vi "副屏设置.vi"() -> ()   [LabVIEW 2016, in "副屏.lvlib"]
uses:
  <vilib>/Utility/config.llb/NI_LVConfig.lvlib
panel:
  in  "屏幕类型":enum16{"HDMI屏", "串口屏"}(ring)
  in  "氟化物":bool caption="氨氮禁用"
  in  "ORP":bool caption="氨氮禁用"
  in  "启用副屏":bool=TRUE caption="氨氮禁用"
  in  "关闭":bool
  in  "底部状态栏显示信息":string="一体化微型水质监测系统"
  in  "流速":bool caption="氨氮禁用"
  in  "瞬时流量":bool caption="氨氮禁用"
  in  "湿度":bool=TRUE caption="氨氮禁用"
  in  "水位":bool caption="氨氮禁用"
  in  "室温":bool=TRUE caption="氨氮禁用"
  in  "CODCr":bool caption="氨氮禁用"
  in  "CODMn":bool caption="氨氮禁用"
  in  "总氮":bool caption="氨氮禁用"
  in  "总磷":bool caption="氨氮禁用"
  in  "氨氮":bool caption="氨氮禁用"
  in  "Turb":bool caption="氨氮禁用"
  in  "Cond":bool caption="氨氮禁用"
  in  "DO":bool caption="氨氮禁用"
  in  "pH":bool caption="氨氮禁用"
  in  "水温":bool caption="氨氮禁用"
  # "副屏显示信息设置"
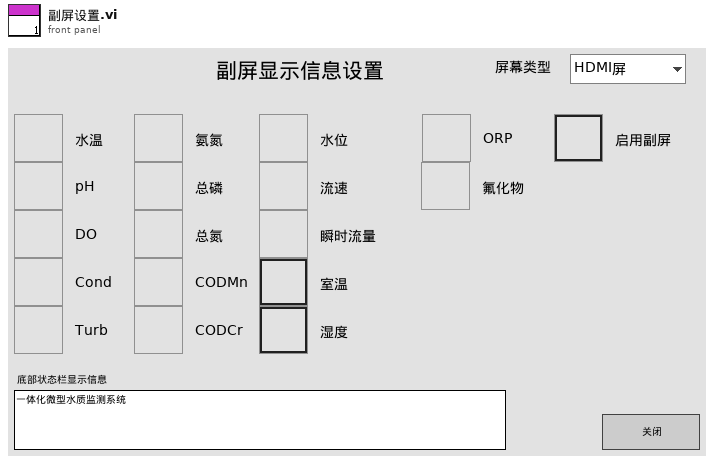
[diagram p1: front panel]
types:
  T1 = typedef "NI_LVConfig.lvlib/Config Data RefNum.ctl" = refnum<k1>
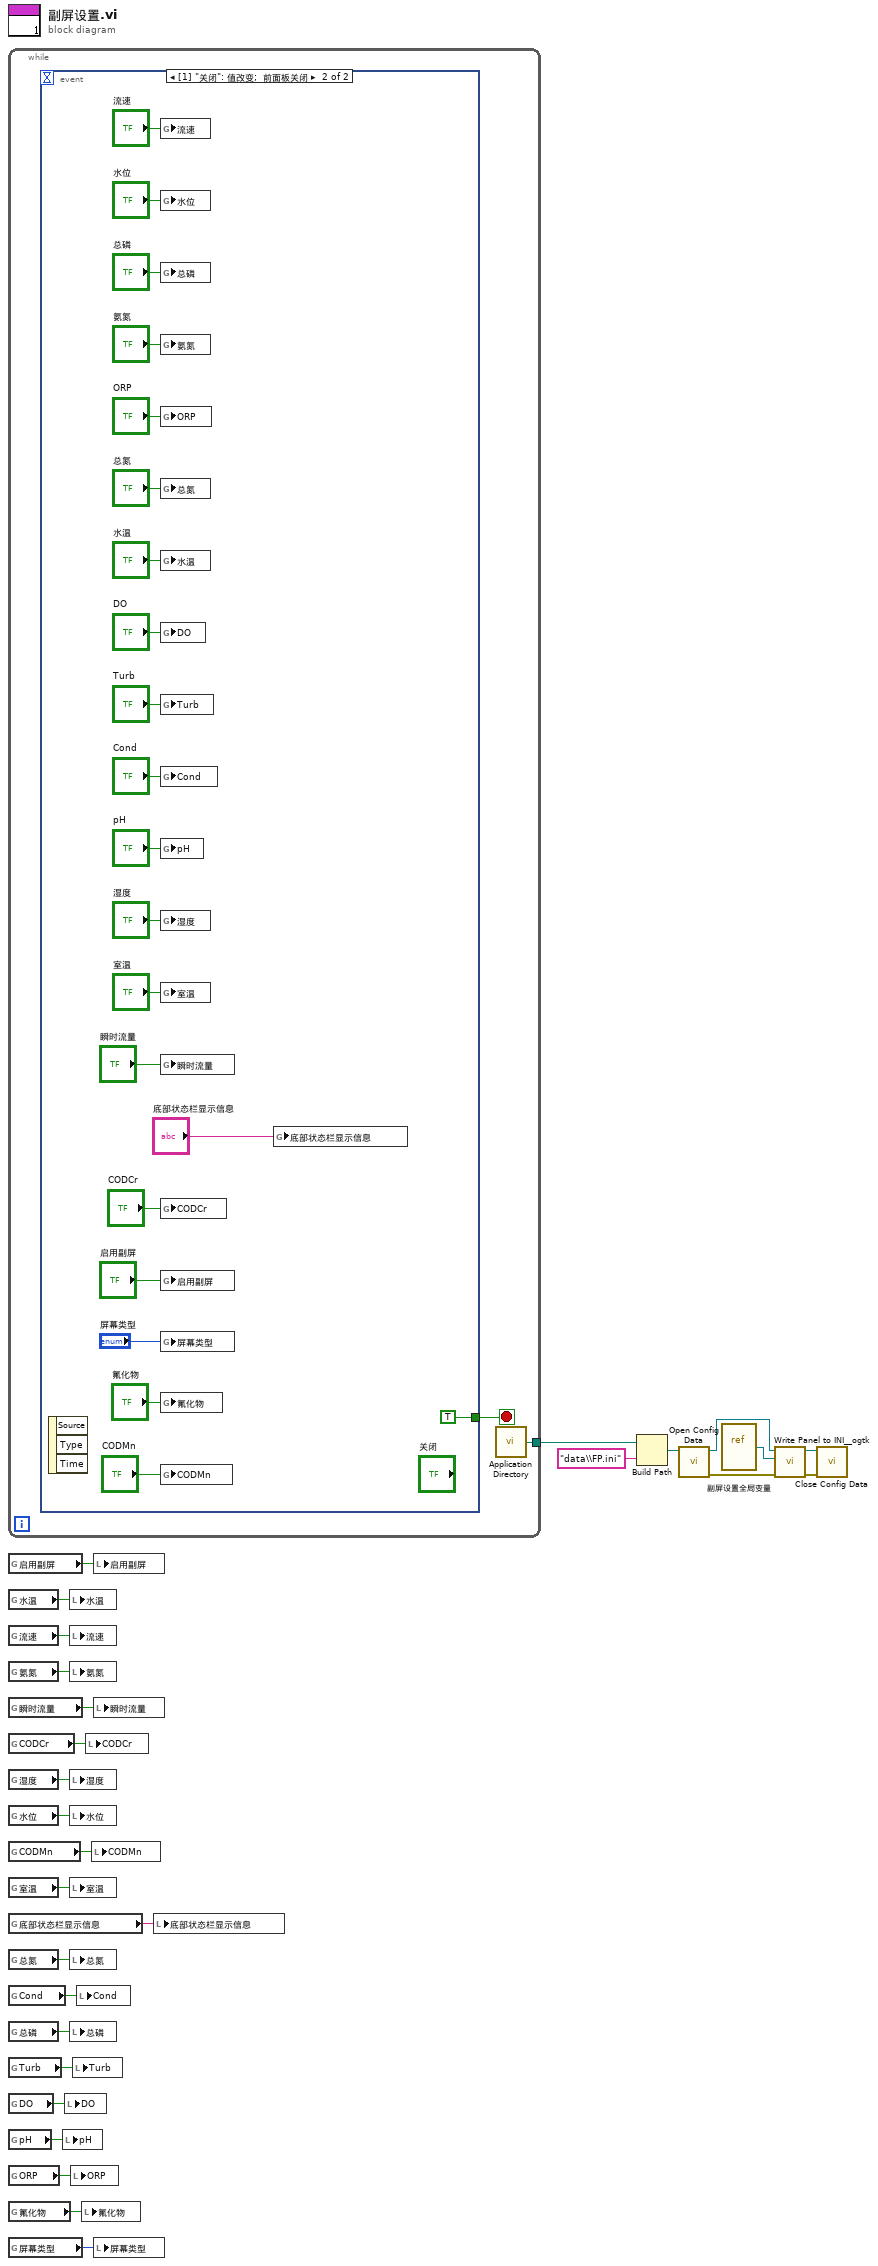
[diagram p0: block diagram]
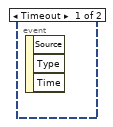
[diagram p2: hidden frame]
diagram:
  n1 = while {
    tunnel: [w29] -> w5
    stop <- w30 stop-if-true
    n2 = event shown="[1] \"关闭\": 值改变;  前面板关闭" {
      selector: _ -> [_ _]
      dyn-events: _ -> [_ _]
      timeout: _ -> [_ _]
      tunnel: [_ TRUE] -> w30
      event Timeout {
        n3 = event-data() -> ()  [unwired: 1 in, 3 out]
      }
      event "关闭": Value Change; Panel Close {
        n4 = event-data() -> ()  [unwired: 1 in, 3 out]
        n5 = global write "副屏设置全局变量.vi" "流速"("流速") -> ()
        n6 = global write "副屏设置全局变量.vi" "水位"("水位") -> ()
        n7 = global write "副屏设置全局变量.vi" "总磷"("总磷") -> ()
        n8 = global write "副屏设置全局变量.vi" "氨氮"("氨氮") -> ()
        n9 = global write "副屏设置全局变量.vi" "ORP"("ORP") -> ()
        n10 = global write "副屏设置全局变量.vi" "总氮"("总氮") -> ()
        n11 = global write "副屏设置全局变量.vi" "水温"("水温") -> ()
        n12 = global write "副屏设置全局变量.vi" "DO"("DO") -> ()
        n13 = global write "副屏设置全局变量.vi" "Turb"("Turb") -> ()
        n14 = global write "副屏设置全局变量.vi" "Cond"("Cond") -> ()
        n15 = global write "副屏设置全局变量.vi" "pH"("pH") -> ()
        n16 = global write "副屏设置全局变量.vi" "湿度"("湿度") -> ()
        n17 = global write "副屏设置全局变量.vi" "室温"("室温") -> ()
        n18 = global write "副屏设置全局变量.vi" "瞬时流量"("瞬时流量") -> ()
        n19 = global write "副屏设置全局变量.vi" "CODCr"("CODCr") -> ()
        n20 = global write "副屏设置全局变量.vi" "启用副屏"("启用副屏") -> ()
        n21 = global write "副屏设置全局变量.vi" "屏幕类型"("屏幕类型") -> ()
        n22 = global write "副屏设置全局变量.vi" "氟化物"("氟化物") -> ()
        n23 = global write "副屏设置全局变量.vi" "CODMn"("CODMn") -> ()
        n24 = global write "副屏设置全局变量.vi" "底部状态栏显示信息"("底部状态栏显示信息") -> ()
      }
    }
    n25 = call <vilib>:"Application Directory.vi"() -> ("Application Directory"=w29:path)
  }
  n26 = global read "副屏设置全局变量.vi" "启用副屏"() -> (w4:bool)
  n27 = global read "副屏设置全局变量.vi" "水温"() -> (w28:bool)
  n28 = global read "副屏设置全局变量.vi" "流速"() -> (w22:bool)
  n29 = global read "副屏设置全局变量.vi" "氨氮"() -> (w27:bool)
  n30 = global read "副屏设置全局变量.vi" "瞬时流量"() -> (w20:bool)
  n31 = global read "副屏设置全局变量.vi" "CODCr"() -> (w26:bool)
  n32 = global read "副屏设置全局变量.vi" "湿度"() -> (w19:bool)
  n33 = global read "副屏设置全局变量.vi" "水位"() -> (w25:bool)
  n34 = global read "副屏设置全局变量.vi" "CODMn"() -> (w24:bool)
  n35 = global read "副屏设置全局变量.vi" "室温"() -> (w16:bool)
  n36 = global read "副屏设置全局变量.vi" "底部状态栏显示信息"() -> (w23:string)
  n37 = global read "副屏设置全局变量.vi" "总氮"() -> (w17:bool)
  n38 = global read "副屏设置全局变量.vi" "Cond"() -> (w21:bool)
  n39 = global read "副屏设置全局变量.vi" "总磷"() -> (w14:bool)
  n40 = global read "副屏设置全局变量.vi" "Turb"() -> (w15:bool)
  n41 = global read "副屏设置全局变量.vi" "DO"() -> (w18:bool)
  n42 = global read "副屏设置全局变量.vi" "pH"() -> (w13:bool)
  n43 = global read "副屏设置全局变量.vi" "ORP"() -> (w3:bool)
  n44 = global read "副屏设置全局变量.vi" "氟化物"() -> (w2:bool)
  n45 = global read "副屏设置全局变量.vi" "屏幕类型"() -> (w1:enum16{"HDMI屏", "串口屏"})
  n46 = local write "pH"(w13) -> ()
  n47 = local write "DO"(w18) -> ()
  n48 = local write "水温"(w28) -> ()
  n49 = local write "流速"(w22) -> ()
  n50 = local write "氨氮"(w27) -> ()
  n51 = local write "湿度"(w19) -> ()
  n52 = local write "水位"(w25) -> ()
  n53 = local write "室温"(w16) -> ()
  n54 = local write "总氮"(w17) -> ()
  n55 = local write "总磷"(w14) -> ()
  n56 = local write "ORP"(w3) -> ()
  n57 = local write "Turb"(w15) -> ()
  n58 = local write "Cond"(w21) -> ()
  n59 = local write "氟化物"(w2) -> ()
  n60 = local write "CODCr"(w26) -> ()
  n61 = local write "CODMn"(w24) -> ()
  n62 = local write "启用副屏"(w4) -> ()
  n63 = local write "瞬时流量"(w20) -> ()
  n64 = local write "屏幕类型"(w1) -> ()
  n65 = local write "底部状态栏显示信息"(w23) -> ()
  n66 = Build Path(base path=w5, name or relative path="data\\FP.ini" ("名称或相对路径")) -> (appended path=w7:path)
  n67 = call <vilib>:"Open Config Data.vi"("configuration file path"=w7) -> ("error out"=w11:errorcluster, "refnum"=w8:T1)  [unwired: 8 in, 1 out]
  n68 = vi-ref "副屏设置全局变量.vi"() -> (w9:refnum<vi>)
  n69 = call <userlib>:"Write Panel to INI__ogtk.vi"("error in (no error)"=w11, "VI ref"=w9, "refnum"=w8) -> ("error out"=w12:errorcluster, "refnum out"=w10:T1)  [unwired: 7 in]
  n70 = call <vilib>:"Close Config Data.vi"("error in (no error)"=w12, "refnum"=w10) -> ()  [unwired: 8 in, 2 out]
